vi "json_number.vi"(5 "text":string, 7 "ch":string, 9 "at":i32, 11 "error in (no error)":errorcluster) -> (4 "number":dbl, 8 "ch out":string, 10 "at out":i32, 15 "error out":errorcluster)   [LabVIEW 2011]
doc: "Parse out a number."
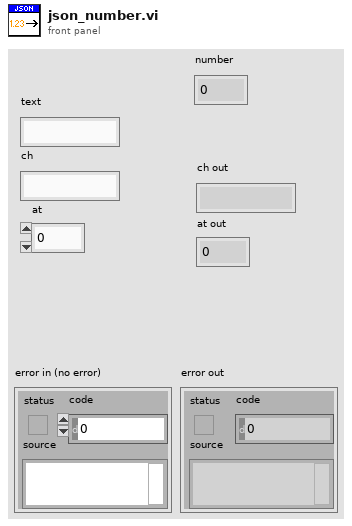
[diagram p1: front panel]
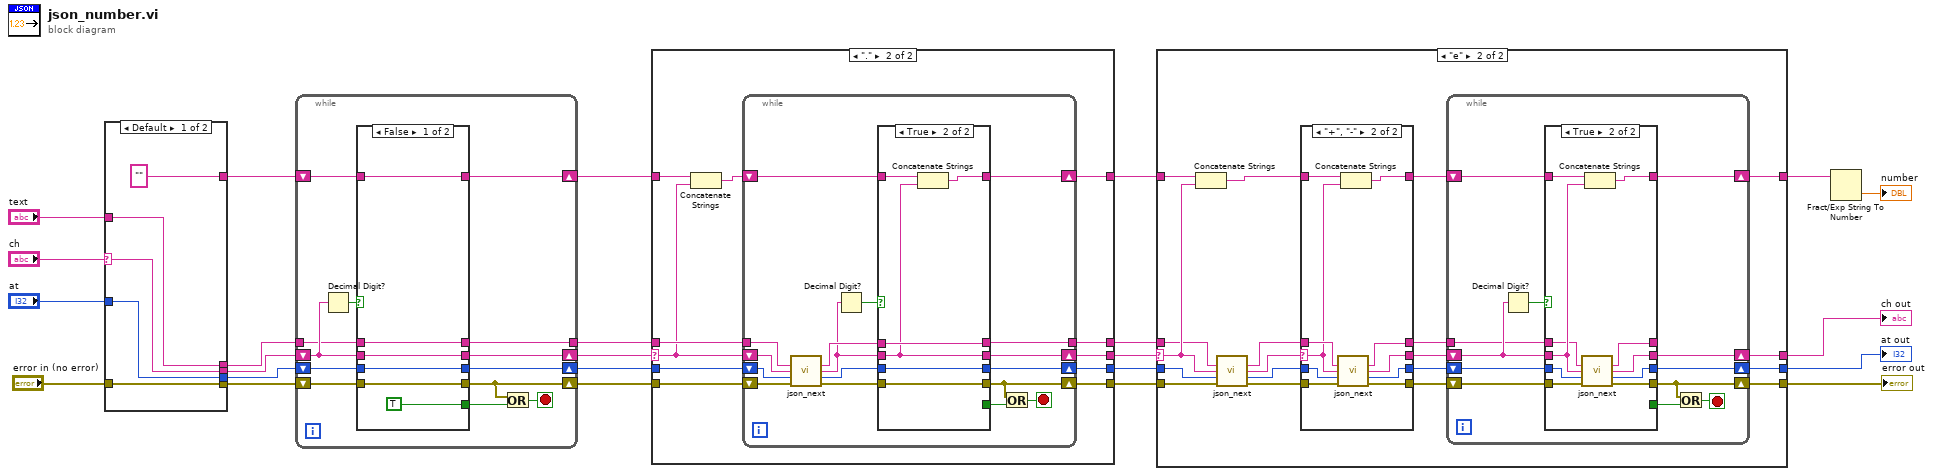
[diagram p0: block diagram]
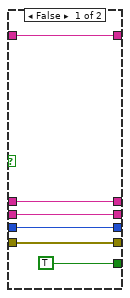
[diagram p4: hidden frame]
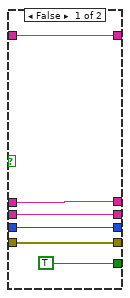
[diagram p6: hidden frame]
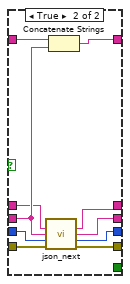
[diagram p7: hidden frame]
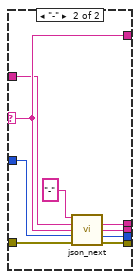
[diagram p8: hidden frame]
diagram:
  n1 = case shown="Default" "ch" {
    selector: "ch" -> [w25 w34]
    tunnel: "error in (no error)" -> [w27 w37]
    tunnel: [w27 w36] -> w13
    tunnel: "at" -> [w26 w35]
    tunnel: "text" -> [w24 w33]
    tunnel: ["" w34] -> w16
    tunnel: [w24 w31] -> w19
    tunnel: [w25 w30] -> w18
    tunnel: [w26 w29] -> w17
    frame Default {
    }
    frame "-" {
      n2 = call "json_next.vi"("c"="-", "text"=w33, "ch"=w34, "at"=w35, "error in (no error)"=w37) -> ("text dup"=w31:string, "ch out"=w30:string, "at out"=w29:i32, "error out"=w36:errorcluster)  [unwired: 7 in]
    }
  }
  n3 = while {
    shift-right: [w40] -> _
    shift-left: w13 -> [w46]
    tunnel: w19 -> [w48]
    shift-right: [w42] -> w15
    shift-left: w18 -> [w49]
    shift-right: [w43] -> w11
    shift-left: w17 -> [w47]
    shift-right: [w44] -> w12
    shift-left: w16 -> [w45]
    tunnel: [w41] -> w14
    stop <- w39 stop-if-true
    n4 = Decimal Digit?(1:w49) -> (0:w50:bool)
    n5 = case shown="False" w50 {
      tunnel: w49 -> [w53 w62]
      tunnel: w48 -> [w51 w61]
      tunnel: w47 -> [w55 w63]
      tunnel: w46 -> [w54 w64]
      tunnel: w45 -> [w56 w66]
      tunnel: [w56 w65] -> w44
      tunnel: [w54 w60] -> w40
      tunnel: [w55 w59] -> w43
      tunnel: [w53 w58] -> w42
      tunnel: [TRUE _] -> w38
      tunnel: [w51 w57] -> w41
      frame False {
      }
      frame True {
        n6 = call "json_next.vi"("text"=w61, "ch"=w62, "at"=w63, "error in (no error)"=w64) -> ("text dup"=w57:string, "ch out"=w58:string, "at out"=w59:i32, "error out"=w60:errorcluster)  [unwired: 8 in]
        n7 = Concatenate Strings(w66, w62) -> (w65:string)
      }
    }
    n8 = Or(x=w40, y=w38) -> (x .or. y?=w39:bool)
  }
  n9 = case shown="\".\"" w15 {
    selector: w15 -> [w69 w73]
    tunnel: w14 -> [w70 w82]
    tunnel: w13 -> [w67 w80]
    tunnel: w12 -> [w71 w75]
    tunnel: w11 -> [w68 w81]
    tunnel: [w70 w79] -> w7
    tunnel: [w69 w78] -> w8
    tunnel: [w68 w77] -> w9
    tunnel: [w67 w76] -> w10
    tunnel: [w71 w72] -> w6
    frame Default {
    }
    frame "." {
      n10 = Concatenate Strings(w75, w73) -> (w74:string)
      n11 = while {
        shift-right: [w85] -> w76
        shift-left: w80 -> [w93]
        tunnel: w82 -> [w89]
        shift-right: [w95] -> w78
        shift-left: w73 -> [w90]
        shift-right: [w96] -> w77
        shift-left: w81 -> [w91]
        shift-right: [w97] -> w72
        shift-left: w74 -> [w98]
        tunnel: [w94] -> w79
        stop <- w83 stop-if-true
        n12 = call "json_next.vi"("text"=w89, "ch"=w90, "at"=w91, "error in (no error)"=w93) -> ("text dup"=w88:string, "ch out"=w87:string, "at out"=w86:i32, "error out"=w92:errorcluster)  [unwired: 8 in]
        n13 = Decimal Digit?(1:w87) -> (0:w99:bool)
        n14 = case shown="True" w99 {
          tunnel: w87 -> [w102 w106]
          tunnel: w88 -> [w100 w109]
          tunnel: w86 -> [w104 w108]
          tunnel: w92 -> [w103 w107]
          tunnel: w98 -> [w105 w111]
          tunnel: [w105 w110] -> w97
          tunnel: [w103 w107] -> w85
          tunnel: [w104 w108] -> w96
          tunnel: [w102 w106] -> w95
          tunnel: [TRUE _] -> w84
          tunnel: [w100 w109] -> w94
          frame False {
          }
          frame True {
            n15 = Concatenate Strings(w111, w106) -> (w110:string)
          }
        }
        n16 = Or(x=w85, y=w84) -> (x .or. y?=w83:bool)
      }
    }
  }
  n17 = case shown="\"e\"" w8 {
    selector: w8 -> [w114 w127]
    tunnel: w7 -> [_ w126]
    tunnel: w10 -> [w112 w123]
    tunnel: w6 -> [w115 w130]
    tunnel: w9 -> [w113 w128]
    tunnel: [w114 w133] -> w3
    tunnel: [w113 w132] -> w2
    tunnel: [w112 w131] -> w1
    tunnel: [w115 w129] -> w5
    frame Default {
    }
    frame "e" {
      n18 = Concatenate Strings(w130, w127) -> (w117:string)
      n19 = call "json_next.vi"("text"=w126, "ch"=w127, "at"=w128) -> ("text dup"=w125:string, "ch out"=w118:string, "at out"=w124:i32)  [unwired: 9 in, 1 out]
      n20 = case shown="\"+\", \"-\"" w118 {
        selector: w118 -> [w134 w139]
        tunnel: w125 -> [w135 w144]
        tunnel: w124 -> [w137 w145]
        tunnel: w123 -> [w136 w146]
        tunnel: w117 -> [w138 w148]
        tunnel: [w138 w147] -> w116
        tunnel: [w136 w143] -> w119
        tunnel: [w137 w142] -> w120
        tunnel: [w134 w141] -> w121
        tunnel: [w135 w140] -> w122
        frame Default {
        }
        frame "+", "-" {
          n21 = call "json_next.vi"("text"=w144, "ch"=w139, "at"=w145, "error in (no error)"=w146) -> ("text dup"=w140:string, "ch out"=w141:string, "at out"=w142:i32, "error out"=w143:errorcluster)  [unwired: 8 in]
          n22 = Concatenate Strings(w148, w139) -> (w147:string)
        }
      }
      n23 = while {
        shift-right: [w150] -> w131
        shift-left: w119 -> [w153]
        tunnel: w122 -> [w154]
        shift-right: [w156] -> w133
        shift-left: w121 -> [w155]
        shift-right: [w157] -> w132
        shift-left: w120 -> [w152]
        shift-right: [w158] -> w129
        shift-left: w116 -> [w159]
        stop <- w149 stop-if-true
        n24 = Decimal Digit?(1:w155) -> (0:w160:bool)
        n25 = case shown="True" w160 {
          tunnel: w155 -> [w163 w172]
          tunnel: w154 -> [w161 w171]
          tunnel: w152 -> [w165 w173]
          tunnel: w153 -> [w164 w174]
          tunnel: w159 -> [w166 w176]
          tunnel: [w166 w175] -> w158
          tunnel: [w164 w170] -> w150
          tunnel: [w165 w169] -> w157
          tunnel: [w163 w168] -> w156
          tunnel: [TRUE _] -> w151
          tunnel: [w161 w167] -> _
          frame False {
          }
          frame True {
            n26 = call "json_next.vi"("text"=w171, "ch"=w172, "at"=w173, "error in (no error)"=w174) -> ("text dup"=w167:string, "ch out"=w168:string, "at out"=w169:i32, "error out"=w170:errorcluster)  [unwired: 8 in]
            n27 = Concatenate Strings(w176, w172) -> (w175:string)
          }
        }
        n28 = Or(x=w150, y=w151) -> (x .or. y?=w149:bool)
      }
    }
  }
  "error out" <- w1
  "ch out" <- w3
  "at out" <- w2
  n29 = Fract/Exp String To Number(string=w5) -> (number=→"number":dbl)  [unwired: 3 in, 1 out]
